vi "Perform Action.vi"(8 "error in (no error)":errorcluster, 10 "Input":variant, 11 "DIO DO PWM DI Meas Freq CFG in":refnum<class "DIO DO PWM DI Meas Freq CFG.lvclass">) -> (0 "error out":errorcluster, 2 "Output":variant, 3 "DIO DO PWM DI Meas Freq CFG out":refnum<class "DIO DO PWM DI Meas Freq CFG.lvclass">)   [LabVIEW 2023, in "DIO DO PWM DI Meas Freq CFG.lvclass"]
uses:
  DIO DO PWM DI Meas Freq CFG.lvclass
  DIO DO PWM DI Meas Freq CFG.lvclass/DIO DO PWM DI Meas Freq CFG.ctl
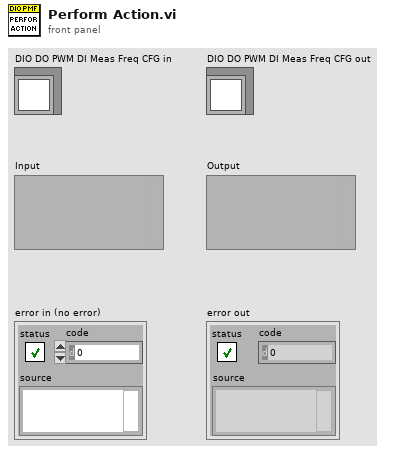
[diagram p1: front panel]
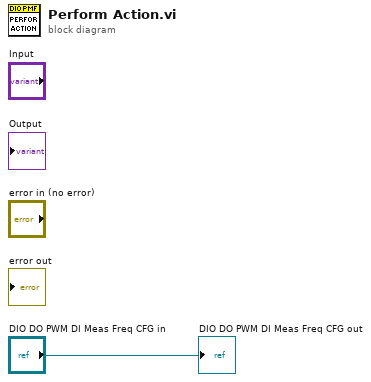
[diagram p0: block diagram]
diagram:
  "DIO DO PWM DI Meas Freq CFG out" <- "DIO DO PWM DI Meas Freq CFG in"
